vi "output.vi"(8 "error in":errorcluster, 10 "output data":T1, 11 "module in":refnum<class "fixed channel tag bus module.lvclass">) -> (0 "error out":errorcluster, 2 "output allocation":T1, 3 "module out":refnum<class "fixed channel tag bus module.lvclass">)   [LabVIEW 2013, in "fixed channel tag bus module.lvclass"]
doc: "Provides an interface for writing data to a module at runtime. While this interface performs no operations, a child should provide an override which may write to any open sessions, references, or interfaces."
uses:
  fixed channel tag bus module.lvclass
  <vilib>/NI/Tag Bus/table/data table.ctl
  <vilib>/NI/Tag Bus/table/data polymorphs/read one/read Double.vi
  <vilib>/NI/Tag Bus/table/data table.lvlib
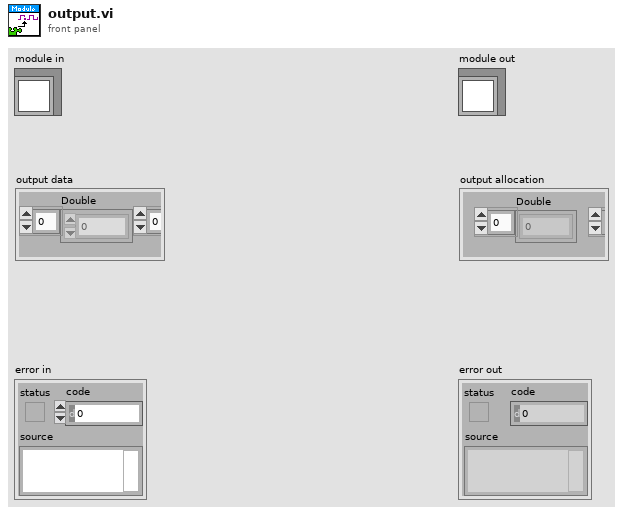
[diagram p1: front panel]
types:
  T1 = typedef "tag bus.lvlib/data table.lvlib/data table.ctl" = cluster{"Double":dbl[], "Single":sgl[], "I64":i64[], "I32":i32[], "I16":i16[], "I8":i8[], "U64":u64[], "U32":u32[], "U16":u16[], "U8":u8[], "Boolean":bool[], "String":string[], "Array of Double":cluster{"DBL Array":dbl[]}[], "Array of Single":cluster{"SGL Array":sgl[]}[], "Array of I64":cluster{"I64 Array":i64[]}[], "Array of I32":cluster{"I32 Array":i32[]}[], "Array of I16":cluster{"I16 Array":i16[]}[], "Array of I8":cluster{"I8 Array":i8[]}[], "Array of U64":cluster{"U64 Array":u64[]}[], "Array of U32":cluster{"U32 Array":u32[]}[], "Array of U16":cluster{"U16 Array":u16[]}[], "Array of U8":cluster{"U8 Array":u8[]}[], "Array of Boolean":cluster{"Boolean Array":bool[]}[], "Array of String":cluster{"String Array":string[]}[]}
  T2 = typedef "fixed channel tag bus module.lvclass/outputs.ctl" = cluster{"placeholder":i32}
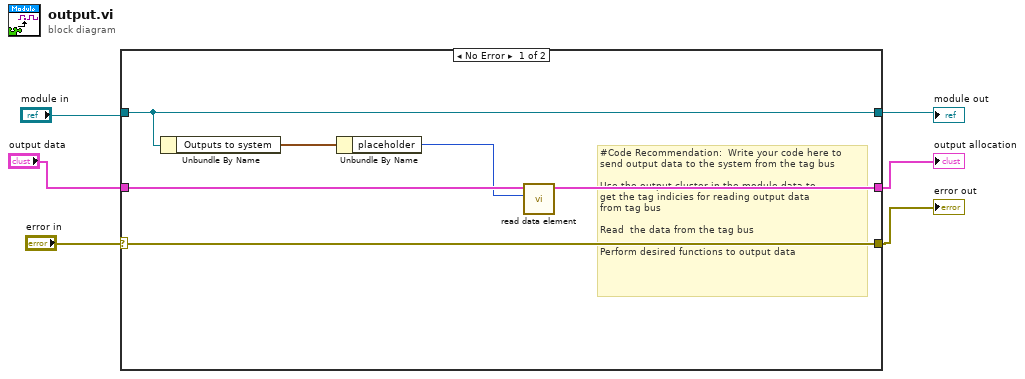
[diagram p0: block diagram]
diagram:
  n1 = case shown="No Error" "error in" {
    selector: "error in" -> [w12 w13]
    tunnel: [w12 w13] -> w1
    tunnel: [w11 w14] -> w3
    tunnel: "output data" -> [w10 w14]
    tunnel: "module in" -> [w9 w15]
    tunnel: [w9 w15] -> w5
    frame No Error {
      # "#Code Recommendation:  Write your code here to\nsend output data to the system from the tag bus\n\nUse the output cluster in the module data to \nget the tag indicies for reading output data\nfrom tag bus\n\nRead  the data from the tag bus\n\nPerform desired functions to output data"
      n2 = Unbundle By Name(w9) -> ("Outputs to system"=w8:T2)
      n3 = Unbundle By Name(w8) -> ("placeholder"=w7:i32)
      n4 = call-poly <vilib>:"read data element.vi"("index"=w7, "data table in"=w10) -> ("data table out"=w11:T1)  [unwired: 8 in, 1 out]
    }
    frame Error {
    }
  }
  "error out" <- w1
  "module out" <- w5
  "output allocation" <- w3
